vi "valesBack.vi"(2 "threshold":dbl, 3 "iPeaksLocation":dbl[](array[numeric]), 4 "filteredSignal":dbl[](array[numeric]), 5 "iPeak":i32) -> (0 "ValesAmplitude":dbl, 1 "iValesLocation":dbl format="%.2f")   [LabVIEW 2011]
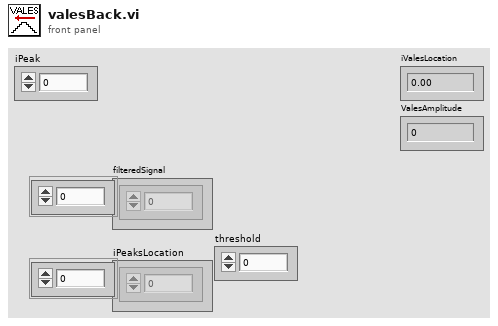
[diagram p1: front panel]
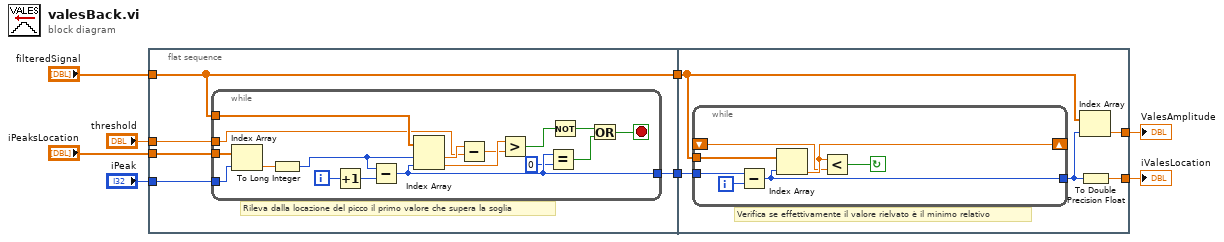
[diagram p0: block diagram]
diagram:
  n1 = flat-sequence {
    tunnel: "filteredSignal" -> [w10]
    tunnel: "iPeaksLocation" -> [w13]
    tunnel: "iPeak" -> [w9]
    tunnel: "threshold" -> [w12]
    tunnel: [w11] -> w4
    tunnel: [w10] -> w3
    tunnel: w4 -> [w35]
    tunnel: w3 -> [w34]
    tunnel: [w31] -> w2
    tunnel: [w32] -> w1
    frame #0 {
      # "Rileva dalla locazione del picco il primo valore che supera la soglia"
      n2 = while {
        tunnel: w10 -> [w28]
        tunnel: w13 -> [w30]
        tunnel: w9 -> [w29]
        tunnel: w12 -> [w22]
        tunnel: [w17] -> w11
        i -> [w27]
        stop <- w19 stop-if-true
        n3 = Index Array(array=w30, index=w29) -> (element=w26:dbl)
        n4 = To Long Integer(number=w26) -> (32bit integer=w24:i32)
        n5 = Increment(x=w27) -> (x+1=w25:i32)
        n6 = Subtract(x=w24, y=w25) -> (x-y=w17:i32)
        n7 = Index Array(array=w28, index #1=w24, index #2=w17) -> (element #1=w23:dbl, element #2=w21:dbl)
        n8 = Subtract(x=w23, y=w22) -> (x-y=w20:dbl)
        n9 = Greater?(x=w21, y=w20) -> (0:w18:bool)
        n10 = Equal?(x=w17, y=0) -> (x = y?=w16:bool)
        n11 = Not(x=w18) -> (.not. x?=w15:bool)
        n12 = Or(x=w15, y=w16) -> (x .or. y?=w19:bool)
      }
    }
    frame #1 {
      # "Verifica se effettivamente il valore rielvato è il minimo relativo"
      n13 = while {
        tunnel: w35 -> [w41]
        tunnel: w34 -> [w42]
        shift-right: [w39] -> _
        shift-left: _ -> [w38]
        tunnel: [w36] -> w33
        i -> [w40]
        stop <- w37 continue-if-true
        n14 = Subtract(x=w41, y=w40) -> (x-y=w36:i32)
        n15 = Index Array(array=w42, index=w36) -> (element=w39:dbl)
        n16 = Less?(x=w39, y=w38) -> (x < y?=w37:bool)
      }
      n17 = Index Array(array=w34, index=w33) -> (element=w32:dbl)
      n18 = To Double Precision Float(number=w33) -> (double precision float=w31:dbl)
    }
  }
  "iValesLocation" <- w2
  "ValesAmplitude" <- w1
